vi "全局变量-35点监测.vi"() -> ()   [LabVIEW 2017]
panel:
  in  "通信单元-改动项引用[]-引用":refnum<vi>
  in  "引用-导出定时配置":refnum<vi>
  in  "引用-累积定时配置":refnum<vi>
  in  "静音延迟 s":u16
  in  "引用-探头信息[]":refnum<vi>
  in  "启用累积功能？":bool
  in  "引用-累积剂量[]":refnum<vi>
  in  "软件版本":string
  in  "调试模式？":bool
  in  "短信通知数据":T1
  in  "屏幕键盘？":bool
  in  "新记录簇":refnum<vi>
  in  "引用-探头属性[]":refnum<vi>
  out "波特率":enum16{"9600", "19200"}(ring)=enum."19200"
  in  "COM口":refnum<visa-resource-name> caption="选择通信端口"
  out "状态类别":string[](array[string])=["全部", "报警", "通信", "设置"]
  out "状态栏-项名[]":refnum<vi>
  in  "最大探头数":i32=32
  in  "停止":bool
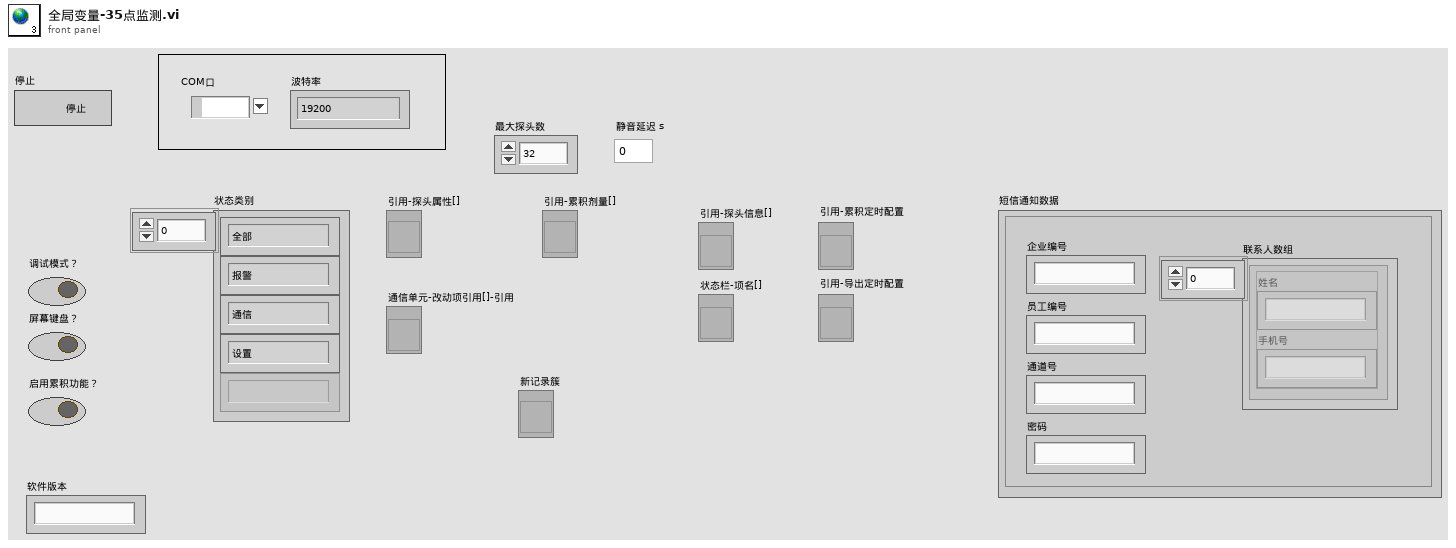
[diagram p1: front panel]
types:
  T1 = cluster{"企业编号":string, "员工编号":string, "通道号":string, "密码":string, "联系人数组":cluster{"姓名":string, "手机号":string}[]}
diagram:
